vi "PPG_ABC.set time.vi"(0 "i ref in":refnum<vi>, 2 "time [us]":dbl, 3 "ms timeout [ms]":i32=10000, 5 "error in (no error)":errorcluster) -> (14 "i ref out":refnum<vi>, 15 "defaultLetter":string, 16 "patternGroup":i32, 17 "timed out":bool, 19 "error out":errorcluster)   [LabVIEW 2014, in "PPG_ABC.lvlib"]
doc: "Recalculates and reloads pattern for given time and default letter - This routine can only by used, after patterns have been loaded using the method \"LoadABC\" and the default letter has been set using the method \"SetDefaultLetter\"."
uses:
  PPG_ABC.lvlib
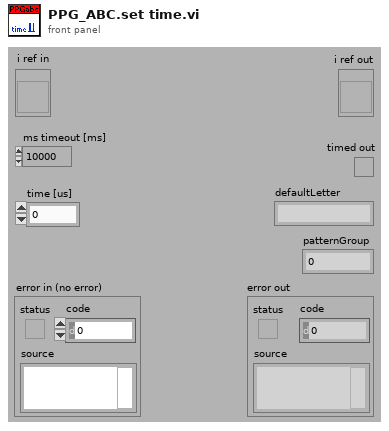
[diagram p1: front panel]
types:
  T1 = typedef "PPG_ABC.lvlib/PPG_ABC.i attribute.ctl" = cluster{"patternGroups":T2[], "defaultLetter":string, "defaultPatternGroup":i32, "PGRunning":T3, "PGRunningID":i32, "pgStarting":T4}
  T2 = typedef "PPG_ABC.lvlib/PPG_ABC.PG_dataType.ctl" = cluster{"PGDevice":string, "rawPatternData":cluster{"triggerCondition":i32, "timeTable":dbl[], "channelTable":string[]}[]}
  T3 = typedef "PPG_ABC.lvlib/PPG_ABC.PG_Running.ctl" = i32
  T4 = typedef "Semaphore RefNum" = refnum<k1>
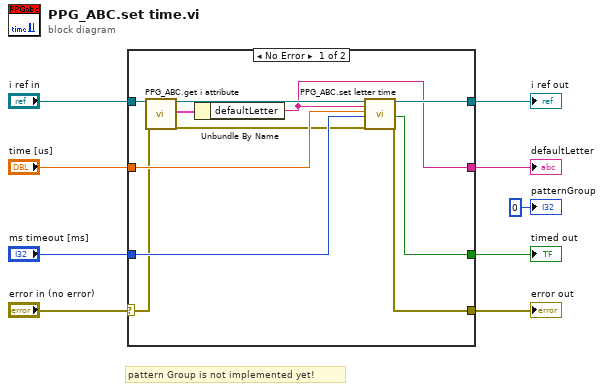
[diagram p0: block diagram]
diagram:
  # "pattern Group is not implemented yet!"
  n1 = case shown="No Error" "error in (no error)" {
    selector: "error in (no error)" -> [w11 w22]
    tunnel: [w14 w22] -> w8
    tunnel: "i ref in" -> [w20 w21]
    tunnel: [w15 w21] -> w6
    tunnel: "ms timeout [ms]" -> [w16 _]
    tunnel: "time [us]" -> [w17 _]
    tunnel: [w13 _] -> w3
    tunnel: [w12 _] -> w2
    frame No Error {
      n2 = call "PPG_ABC.get i attribute.vi"("i ref in"=w20, "error in (no error)"=w11) -> ("i ref out"=w18:refnum<vi>, "i attribute"=w19:T1, "error out"=w10:errorcluster)  [unwired: 15 in]
      n3 = Unbundle By Name(w19) -> ("defaultLetter"=w12:string)
      n4 = call "PPG_ABC.set letter time.vi"("i ref in"=w18, "letter"=w12, "time [us]"=w17, "ms timeout [ms]"=w16, "error in (no error)"=w10) -> ("i ref out"=w15:refnum<vi>, "timed out"=w13:bool, "error out"=w14:errorcluster)  [unwired: 12 in]
    }
    frame Error {
    }
  }
  "error out" <- w8
  "i ref out" <- w6
  "timed out" <- w3
  "defaultLetter" <- w2
  "patternGroup" <- 0 ("patternGroup")
